vi "disconnect.vi"(8 "error in (no error)":errorcluster, 11 "SAL_Listener in":refnum<class "SAL_Listener.lvclass">) -> (0 "error out":errorcluster, 3 "SAL_Listener out":refnum<class "SAL_Listener.lvclass">)   [LabVIEW 2016, in "SAL_Listener.lvclass"]
uses:
  SAL_Listener.lvclass
  SALLV_dome/SALLV_dome.lvlib
  SALLV_domeADB/SALLV_domeADB.lvlib
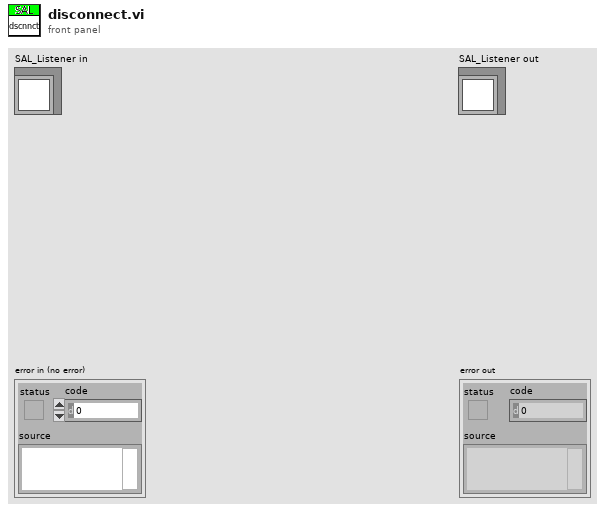
[diagram p1: front panel]
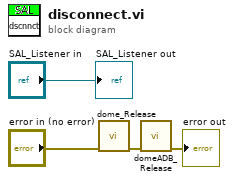
[diagram p0: block diagram]
diagram:
  n1 = call "dome_Release.vi"("error in (no error)"="error in (no error)") -> ("error out"=w2:errorcluster)  [unwired: 9 in, 1 out]
  n2 = call "domeADB_Release.vi"("error in (no error)"=w2) -> ("error out"=→"error out":errorcluster)  [unwired: 9 in, 1 out]
  "SAL_Listener out" <- "SAL_Listener in"
